vi "Create Arbitrary Waveform.vi"(6 "Waveform Label (Default)":string="Default", 7 "Waveform Slot (1: Slot 1)":i32(ring)=1 items=["Slot 1"=1, "Slot 2"=2, "Slot 3"=3, "Slot 4"=4], 8 "error in (no error)":errorcluster, 9 "Number Of Points (100)":i32=100, 10 "Waveform Function (0: Sine)":i32(ring) items=["Sine", "Square", "Pulse", "Ramp", "Noise"], 11 "VISA resource name":refnum<visa-resource-name>) -> (0 "error out":errorcluster, 3 "VISA resource name out":refnum<visa-resource-name>)   [LabVIEW 2016, in "Tektronix DPO MSO 2000 4000 Series.lvlib"]
doc: "Configures the waveform label and generates the arbitrary waveform function.\n\n<B>Notes:</B>\n(1) This VI is available for MDO3000 Series only.\n\n(2) Requires the MDO3AFG option to be installed."
uses:
  Tektronix DPO MSO 2000 4000 Series.lvlib
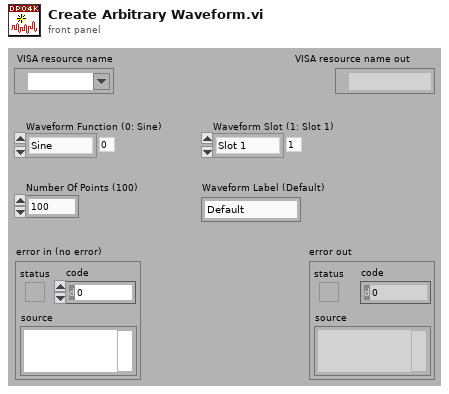
[diagram p1: front panel]
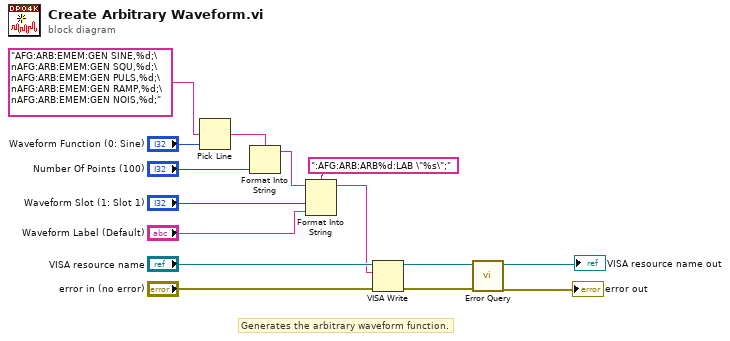
[diagram p0: block diagram]
diagram:
  # "Generates the arbitrary waveform function."
  n1 = Pick Line(multi-line string="AFG:ARB:EMEM:GEN SINE,%d;\nAFG:ARB:EMEM:GEN SQU,%d;\nAFG:ARB:EMEM:GEN PULS,%d;\nAFG:ARB:EMEM:GEN RAMP,%d;\nAFG:ARB:EMEM:GEN NOIS,%d;", line index="Waveform Function (0: Sine)") -> (output string=w5:string)  [unwired: 1 in]
  n2 = Format Into String(format string=w5, "Number Of Points (100)") -> (resulting string=w3:string)  [unwired: 2 in, 1 out]
  n3 = Format Into String(format string=":AFG:ARB:ARB%d:LAB \"%s\";", initial string=w3, "Waveform Slot (1: Slot 1)", "Waveform Label (Default)") -> (resulting string=w2:string)  [unwired: 1 in, 1 out]
  n4 = VISA Write(VISA resource name="VISA resource name", write buffer=w2, error in (no error)="error in (no error)") -> (VISA resource name out=w12:refnum<visa-resource-name>, error out=w11:errorcluster)  [unwired: 1 out]
  n5 = call "Error Query.vi"("error in (no error)"=w11, "VISA resource name"=w12) -> ("error out"=→"error out":errorcluster, "VISA resource name out"=→"VISA resource name out":refnum<visa-resource-name>)  [unwired: 6 in, 2 out]
